vi "Calculate Waveform.vi"(6 "Channel":u8, 7 "Head <JSON>":string, 8 "error in (no error)":errorcluster, 9 "Points":i16[](array[numeric]), 10 "Acquisition Time":timestamp, 11 "OWON SDS1022 in":refnum<class "SDS1000 Base CFG.lvclass">) -> (0 "error out":errorcluster, 2 "Waveform Graph":waveform(dbl)(graph), 3 "OWON SDS1022 out":refnum<class "SDS1000 Base CFG.lvclass">)   [LabVIEW 2023, in "OWON SDS1022.lvlib" / "SDS1000 Base CFG.lvclass"]
uses:
  SDS1000 Base CFG.lvclass
  SDS1000 Base CFG.lvclass/SDS1000 Base CFG.ctl
  5ff70b4c-a951-438e-aa90-247ca6a210be.vi
  b003ad20-f1c5-4d81-8556-46127c723614.vi
  <vilib>/JDP Science/JSONtext/Find Item.vi
  <vilib>/JDP Science/JSONtext/Next JSON Value.vi
  <vilib>/JDP Science/JSONtext/String Subset.vi
  <vilib>/JDP Science/JSONtext/Parsing/Advance past next JSON Value (inlined COPY).vi
  <vilib>/JDP Science/JSONtext/Parsing/Advance past whitespace.vi
  <vilib>/JDP Science/JSONtext/Parsing/Advance past String.vi
  <vilib>/JDP Science/JSONtext/Parsing/Advance past Number.vi
  <vilib>/JDP Science/JSONtext/Parsing/Advance past Line Ending.vi
  <vilib>/JDP Science/JSONtext/Parsing/Parse Full Path or Item Name.vi
  <vilib>/JDP Science/JSONtext/Parsing/Advance past Array.vi
  <vilib>/JDP Science/JSONtext/Parsing/Advance past Object.vi
  <vilib>/JDP Science/JSONtext/support/Error Cluster From Code.vi
  <vilib>/JDP Science/JSONtext/Offset/Find Item Locations by Path.vi
  <vilib>/JDP Science/JSONtext/JSON text to Variant.vi
  <vilib>/Utility/error.llb/Error Cluster From Error Code.vi
  <vilib>/JDP Science/JSONtext/LVClass Serializer/JSONtext LVClass Serializer.lvclass
  <vilib>/ErrorRing/Error Ring.xnode
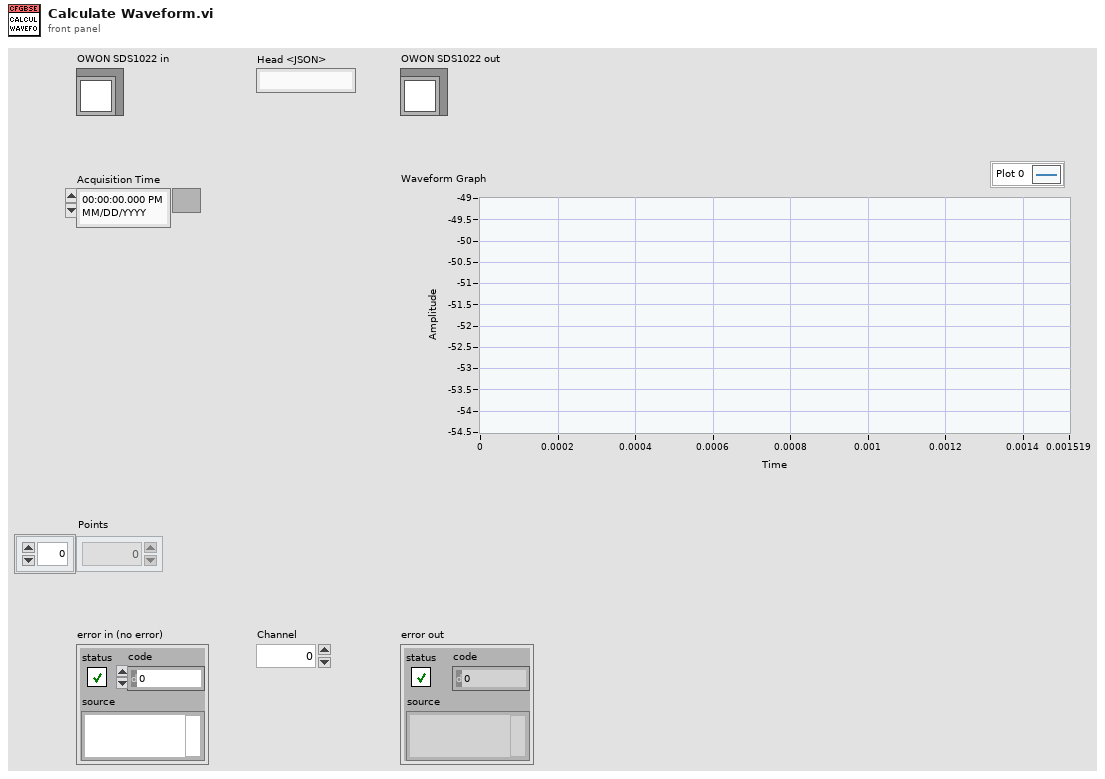
[diagram p1: front panel]
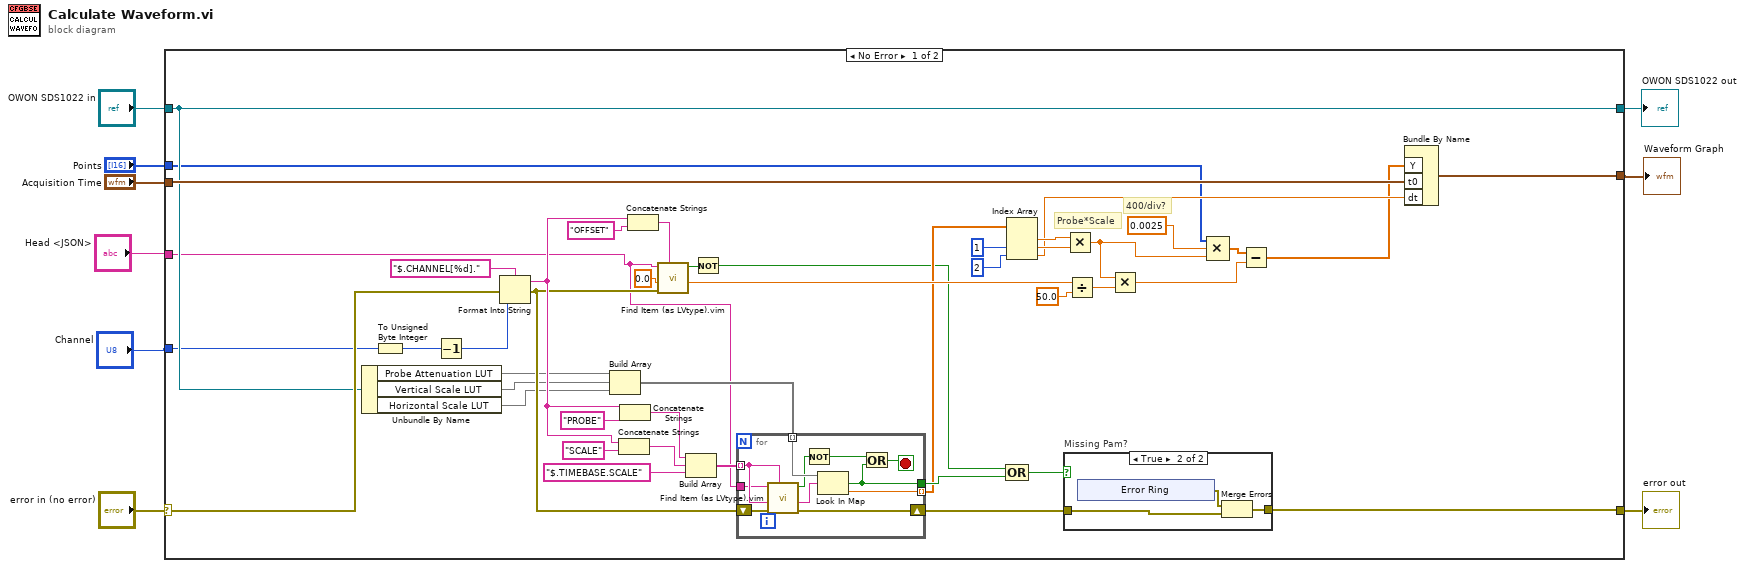
[diagram p0: block diagram]
diagram:
  n1 = case shown="No Error" "error in (no error)" {
    selector: "error in (no error)" -> [w54 w76]
    tunnel: [w52 w76] -> w8
    tunnel: [w20 w75] -> w6
    tunnel: "OWON SDS1022 in" -> [w20 w75]
    tunnel: "Points" -> [w10 _]
    tunnel: "Acquisition Time" -> [w51 _]
    tunnel: [w21 _] -> w3
    tunnel: "Channel" -> [w19 _]
    tunnel: "Head <JSON>" -> [w18 _]
    frame No Error {
      # "Probe*Scale"
      # "400/div?"
      n2 = Unbundle By Name(w20) -> ("Probe Attenuation LUT"=w34:map{string, dbl}, "Vertical Scale LUT"=w33:map{string, dbl}, "Horizontal Scale LUT"=w32:map{string, dbl})
      n3 = To Unsigned Byte Integer(number=w19) -> (unsigned 8bit integer=w40:u8)
      n4 = Decrement(x=w40) -> (x-1=w39:u8)
      n5 = Format Into String(format string="$.CHANNEL[%d].", error in=w54, w39) -> (resulting string=w45:string, error out=w43:errorcluster)  [unwired: 1 in]
      n6 = Build Array(w34, w33, w32) -> (w31:map{string, dbl}[])
      n7 = Concatenate Strings(w45, "SCALE" ("$Path or Item Name")) -> (w36:string)
      n8 = Concatenate Strings(w45, "PROBE" ("$Path or Item Name")) -> (w35:string)
      n9 = Concatenate Strings(w45, "OFFSET" ("$Path or Item Name")) -> (w48:string)
      n10 = call "Find Item (as LVtype).vim"("$Path or Item Name"=w48, "error in (no error)"=w43, "Data Type and Default Value"=0.0, "JSON"=w18) -> ("Data"=w42:dbl, "Found"=w23:bool)  [unwired: 4 in, 2 out]
      n11 = Build Array(w35, w36, "$.TIMEBASE.SCALE" ("$Path or Item Name")) -> (w37:string[])
      n12 = Not(x=w23) -> (.not. x?=w22:bool)
      n13 = for {
        tunnel: [w63] -> w29 mode=indexing
        tunnel: w37 -> [w62] mode=indexing
        tunnel: w18 -> [w60]
        shift-right: [w64] -> w53
        shift-left: w43 -> [w61]
        tunnel: w31 -> [w59] mode=indexing
        tunnel: [w55] -> w30
        stop <- w56 stop-if-true
        n14 = call "Find Item (as LVtype).vim"("$Path or Item Name"=w62, "error in (no error)"=w61, "Data Type and Default Value"=w62, "JSON"=w60) -> ("error out"=w64:errorcluster, "Data"=w65:string, "Found"=w58:bool)  [unwired: 4 in, 1 out]
        n15 = Not(x=w58) -> (.not. x?=w57:bool)
        n16 = Look In Map(map=w59, key=w65) -> (key not found?=w55:bool, value=w63:dbl)  [unwired: 1 in]
        n17 = Or(x=w57, y=w55) -> (x .or. y?=w56:bool)
      }
      n18 = Compound Arithmetic op=OR(w22, w30) -> (w50:bool)
      n19 = Index Array(array=w29, index #2=1 ("index"), index #3=2 ("index")) -> (element #1=w28:dbl, element #2=w26:dbl, element #3=w24:dbl)  [unwired: 1 in]
      n20 = case "Missing Pam?" shown="True" w50 {
        tunnel: w53 -> [w66 w68]
        tunnel: [w66 w67] -> w52
        frame False {
        }
        frame True {
          n21 = xnode "Error Ring"() -> ("error out"=w69:errorcluster)
          n22 = Merge Errors(w69, w68) -> (w67:errorcluster)
        }
      }
      n23 = Multiply(x=w28, y=w26) -> (x*y=w13:dbl)
      n24 = Divide(x=w42, y=50.0) -> (x/y=w14:dbl)
      n25 = Multiply(x=w13, y=w14) -> (x*y=w12:dbl)
      n26 = Compound Arithmetic op=MULTIPLY(w10, 0.0025, w13) -> (w17:dbl[])
      n27 = Subtract(x=w17, y=w12) -> (x-y=w11:dbl[])
      n28 = Bundle By Name("Y"=w11, "t0"=w51, "dt"=w24) -> (w21:waveform(dbl))  [unwired: 1 in]
    }
    frame Error {
    }
  }
  "error out" <- w8
  "OWON SDS1022 out" <- w6
  "Waveform Graph" <- w3
